vi "(SubVI) Smooth QPD data and Get its position_YCC.vi"(4 "Filter type":T1(ring), 5 "Initial position (um)":dbl, 6 "Avg points":i32, 7 "scan rate  (um/s)":dbl=2.0 format="%.3f", 8 "Sampling rate (Hz)":dbl=20000.0, 9 "QPD data":dbl[](array[numeric]), 11 "Direction\nT=+ \nF=-":bool) -> (1 "Filtered QPD data":dbl[](array[numeric]), 2 "Filtered Stage Array":dbl[](array[numeric]), 3 "Raw Stage Array":dbl[](array[numeric]))   [LabVIEW 2014]
panel:
  out "XY Graph":cluster{dbl[], dbl[]}[](graph)
  out "Sampling rate after filtering (Hz)":dbl
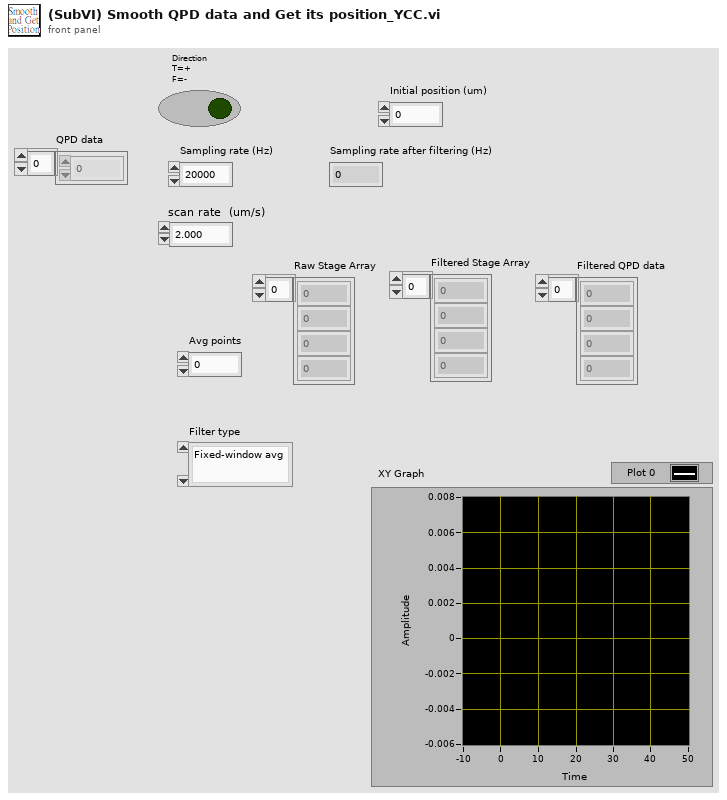
[diagram p1: front panel]
types:
  T1 = enum16{"Fixed-window avg", "Moving-window avg", "F+S-window avg", "S-G filter", "Fixed-window Median", "Moving-window Median "}
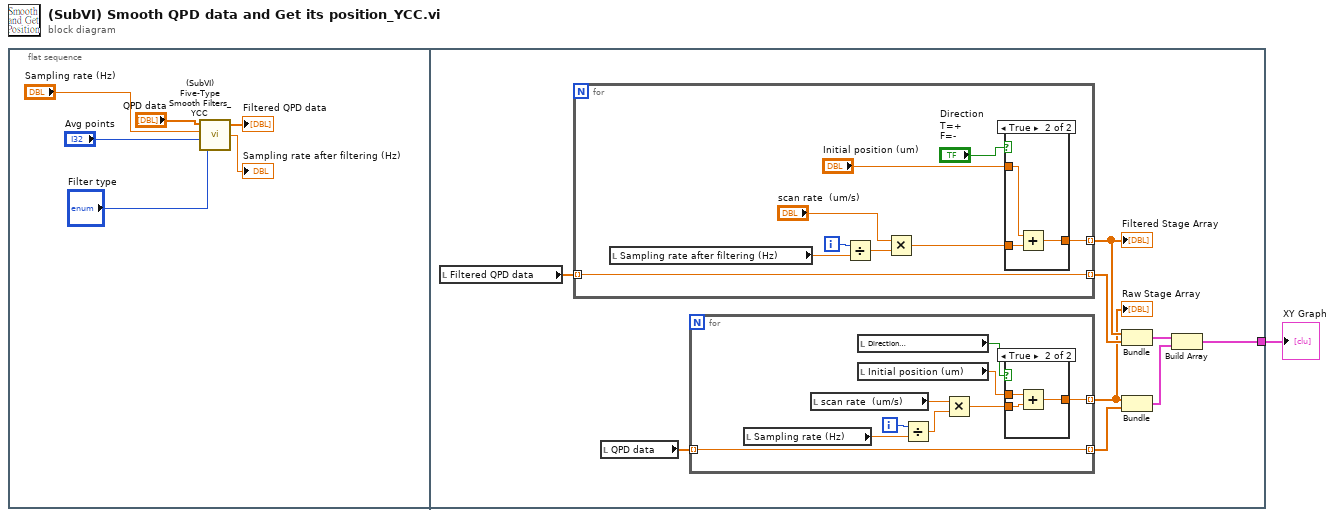
[diagram p0: block diagram]
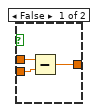
[diagram p2: hidden frame]
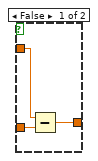
[diagram p3: hidden frame]
diagram:
  n1 = flat-sequence {
    tunnel: [w10] -> w1
    frame #0 {
      n2 = call "(SubVI) Five-Type Smooth Filters_YCC.vi"("Filter type"="Filter type", "Avg points"="Avg points", "Sampling rate (Hz)"="Sampling rate (Hz)", "QPD data"="QPD data") -> ("Sampling rate after filtering (Hz)"=→"Sampling rate after filtering (Hz)":dbl, "Filtered QPD data"=→"Filtered QPD data":dbl[])  [unwired: 1 in]
    }
    frame #1 {
      n3 = local read "Filtered QPD data"() -> (w9:dbl[])
      n4 = for {
        tunnel: w9 -> [w38] mode=indexing
        tunnel: [w38] -> w16 mode=indexing
        tunnel: [w33] -> w15 mode=indexing
        i -> [w40]
        n5 = local read "Sampling rate after filtering (Hz)"() -> (w32:dbl)
        n6 = Divide(x=w40, y=w32) -> (x/y=w39:dbl)
        n7 = Multiply(x="scan rate  (um/s)", y=w39) -> (x*y=w34:dbl)
        n8 = case shown="True" "Direction\nT=+ \nF=-" {
          tunnel: "Initial position (um)" -> [w43 w46]
          tunnel: w34 -> [w42 w45]
          tunnel: [w41 w44] -> w33
          frame False {
            n9 = Subtract(x=w43, y=w42) -> (x-y=w41:dbl)
          }
          frame True {
            n10 = Add(x=w46, y=w45) -> (x+y=w44:dbl)
          }
        }
      }
      "Filtered Stage Array" <- w15
      n11 = local read "QPD data"() -> (w14:dbl[])
      n12 = for {
        tunnel: w14 -> [w23] mode=indexing
        tunnel: [w23] -> w13 mode=indexing
        tunnel: [w21] -> w8 mode=indexing
        i -> [w25]
        n13 = local read "Sampling rate (Hz)"() -> (w20:dbl)
        n14 = local read "scan rate  (um/s)"() -> (w19:dbl)
        n15 = local read "Direction\nT=+ \nF=-"() -> (w17:bool)
        n16 = local read "Initial position (um)"() -> (w18:dbl)
        n17 = Divide(x=w25, y=w20) -> (x/y=w24:dbl)
        n18 = Multiply(x=w19, y=w24) -> (x*y=w22:dbl)
        n19 = case shown="True" w17 {
          tunnel: w18 -> [w28 w31]
          tunnel: w22 -> [w27 w30]
          tunnel: [w26 w29] -> w21
          frame False {
            n20 = Subtract(x=w28, y=w27) -> (x-y=w26:dbl)
          }
          frame True {
            n21 = Add(x=w31, y=w30) -> (x+y=w29:dbl)
          }
        }
      }
      "Raw Stage Array" <- w8
      n22 = Bundle(w15, w16) -> (w12:cluster{dbl[], dbl[]})  [unwired: 1 in]
      n23 = Bundle(w8, w13) -> (w11:cluster{dbl[], dbl[]})  [unwired: 1 in]
      n24 = Build Array(w12, w11) -> (w10:cluster{dbl[], dbl[]}[])
    }
  }
  "XY Graph" <- w1
